vi "Controller.vi"(0 "Process Variable":dbl, 1 "Pressure Controller Dynamics":T1={"Proportional Gain Positive"=2e-08, "Proportional Gain Negative"=8e-08}, 2 "Manual Control":bool, 3 "On/Off":bool, 5 "Pressure Set Point":dbl, 7 "Manual Signals":cluster{"Positive":dbl, "Negative":dbl}, 9 "Branch IN":bool, 11 "Previous Signals":cluster{"Positive":dbl, "Negative":dbl}, 12 "Minimum Value":dbl=0.5 caption="Min Value" format="%0.2f", 13 "Maximum Value":dbl=1.0 caption="Max Value" format="%0.2f") -> (4 "External Signals":cluster{"Positive":dbl, "Negative":dbl}, 8 "Branch OUT":bool, 10 "Valves":bool, 15 "Internal Signals":cluster{"Positive":dbl, "Negative":dbl})   [LabVIEW 2012, in "Pressure Regulator Controller.lvlib"]
uses:
  Pressure Regulator Controller.lvlib
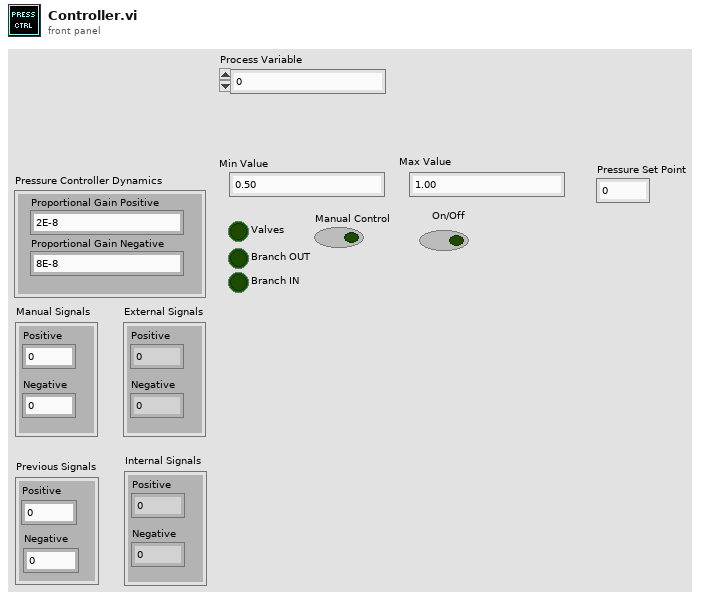
[diagram p1: front panel]
types:
  T1 = cluster{"Proportional Gain Positive":dbl, "Proportional Gain Negative":dbl}
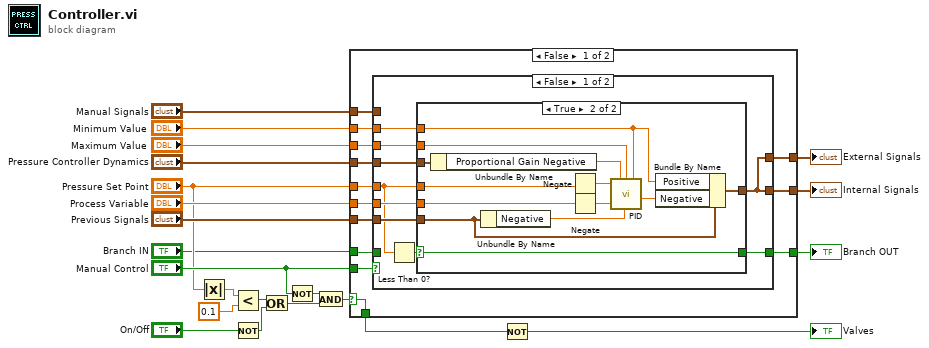
[diagram p0: block diagram]
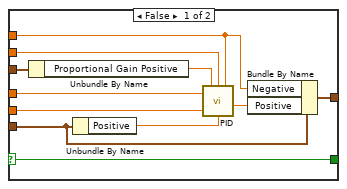
[diagram p2: hidden frame]
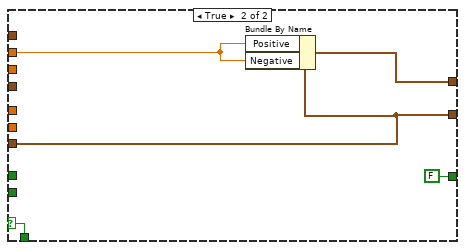
[diagram p4: hidden frame]
diagram:
  n1 = Absolute Value(x="Pressure Set Point") -> (abs(x)=w22:dbl)
  n2 = Less?(x=w22, y=0.1) -> (x < y?=w20:bool)
  n3 = Not(x="On/Off") -> (.not. x?=w2:bool)
  n4 = Or(x=w20, y=w2) -> (x .or. y?=w17:bool)
  n5 = Not(x="Manual Control") -> (.not. x?=w18:bool)
  n6 = And(x=w18, y=w17) -> (x .and. y?=w7:bool)
  n7 = case shown="False" w7 {
    selector: w7 -> [w28 w76]
    tunnel: "Previous Signals" -> [w35 w73]
    tunnel: [w26 w74] -> w15
    tunnel: [w25 w73] -> w14
    tunnel: "Minimum Value" -> [w33 w75]
    tunnel: "Pressure Set Point" -> [w34 _]
    tunnel: "Maximum Value" -> [w32 _]
    tunnel: "Pressure Controller Dynamics" -> [w31 _]
    tunnel: "Process Variable" -> [w30 _]
    tunnel: "Manual Signals" -> [w29 _]
    tunnel: [w28 w76] -> w8
    tunnel: "Manual Control" -> [w27 _]
    tunnel: [w24 FALSE ("Branch IN")] -> w4
    tunnel: "Branch IN" -> [w23 _]
    frame False {
      n8 = case shown="False" w27 {
        tunnel: w35 -> [w44 w70]
        tunnel: w34 -> [w38 _]
        tunnel: w33 -> [w42 _]
        tunnel: w32 -> [w41 _]
        tunnel: w31 -> [w40 _]
        tunnel: w30 -> [w39 _]
        tunnel: w29 -> [_ w71]
        tunnel: [w37 w71] -> w26
        tunnel: [w37 w70] -> w25
        tunnel: [w36 w69] -> w24
        tunnel: w23 -> [_ w69]
        frame False {
          n9 = Less Than 0?(x=w38) -> (x < 0?=w43:bool)
          n10 = case shown="True" w43 {
            selector: w43 -> [w45 w56]
            tunnel: w38 -> [w54 w68]
            tunnel: w39 -> [w55 w67]
            tunnel: w42 -> [w46 w57]
            tunnel: w41 -> [w53 w64]
            tunnel: w44 -> [w48 w59]
            tunnel: w40 -> [w51 w61]
            tunnel: [w49 w60] -> w37
            tunnel: [w45 w56] -> w36
            frame False {
              n11 = Unbundle By Name(w51) -> ("Proportional Gain Positive"=w50:dbl)
              n12 = Unbundle By Name(w48) -> ("Positive"=w52:dbl)
              n13 = call "PID.vi"("Set Point"=w54, "Min output value"=w46, "Max output value"=w53, "Process Variable"=w55, "Previous Output"=w52, "Proportional Gain"=w50) -> ("Output"=w47:dbl)  [unwired: 7 in, 2 out]
              n14 = Bundle By Name(cluster=w48, "Negative"=w46, "Positive"=w47) -> (w49:cluster{"Positive":dbl, "Negative":dbl})
            }
            frame True {
              n15 = Unbundle By Name(w61) -> ("Proportional Gain Negative"=w62:dbl)
              n16 = Unbundle By Name(w59) -> ("Negative"=w63:dbl)
              n17 = Negate(x=w68) -> (-x=w66:dbl)
              n18 = Negate(x=w67) -> (-x=w65:dbl)
              n19 = call "PID.vi"("Set Point"=w66, "Min output value"=w57, "Max output value"=w64, "Process Variable"=w65, "Previous Output"=w63, "Proportional Gain"=w62) -> ("Output"=w58:dbl)  [unwired: 7 in, 2 out]
              n20 = Bundle By Name(cluster=w59, "Positive"=w57, "Negative"=w58) -> (w60:cluster{"Positive":dbl, "Negative":dbl})
            }
          }
        }
        frame True {
        }
      }
    }
    frame True {
      n21 = Bundle By Name(cluster=w73, "Positive"=w75, "Negative"=w75) -> (w74:cluster{"Positive":dbl, "Negative":dbl})
    }
  }
  "External Signals" <- w15
  "Internal Signals" <- w14
  "Branch OUT" <- w4
  n22 = Not(x=w8) -> (.not. x?=→"Valves":bool)
